vi "ZMQ Send command string input.vi"(4 "Int args":map{string, i32}(c390), 5 "String args":map{string, string}(c390), 6 "Bool args":map{string, bool}(c390), 7 "DBL args":map{string, dbl}(c390), 8 "error in":errorcluster, 9 "Command":string, 10 "Instrument":string, 11 "socket in":refnum<class "zmq_socket.lvclass">) -> (0 "error out":errorcluster, 1 "Standalone":bool, 2 "Recieved message":string=" INSTRUCTIONS:\r\rNormal Use:  When using subVIs that incorporate the error in/error out (or error I/O) structure, place this handler where you want to inform the user of an error, typically at the end of the I/O data path, as the last action of the program.  If the error in error? is ERROR, the handler creates a message describing the error and its source.  If the type of dialog = 1 (default), the message is displayed to the user, who can only acknowedge it.  If the type = 2, the user can acknowledge the message or abort execution; aborting a program with active I/O is not recommended.  If the type = 0, no message is displayed; this is used to process the error programmatically, and the error out cluster elements are wired to individual terminals for that reason.  \r\rOther Use:\n\r\nlocal testing.  To test the error code of a subVI or function that does not have the error I/O structure, you can wire its error code and a source string to the local error code and error source inputs.  If error in error? indicates no error and error code is not equal to 0, the local code and source are substituted for the error in values, and error? is set TRUE (ERROR).", 3 "socket out":refnum<class "zmq_socket.lvclass">)   [LabVIEW 2022 SP3]
uses:
  <vilib>/addons/zeromq/zmq_socket.lvclass
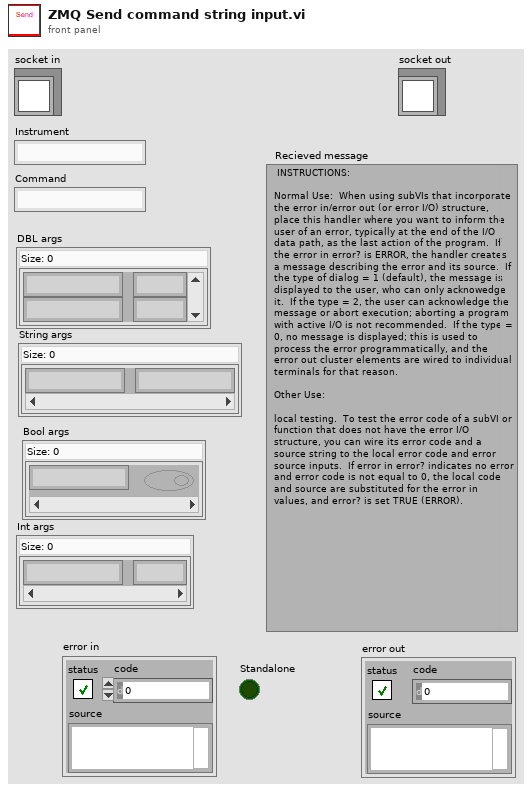
[diagram p1: front panel]
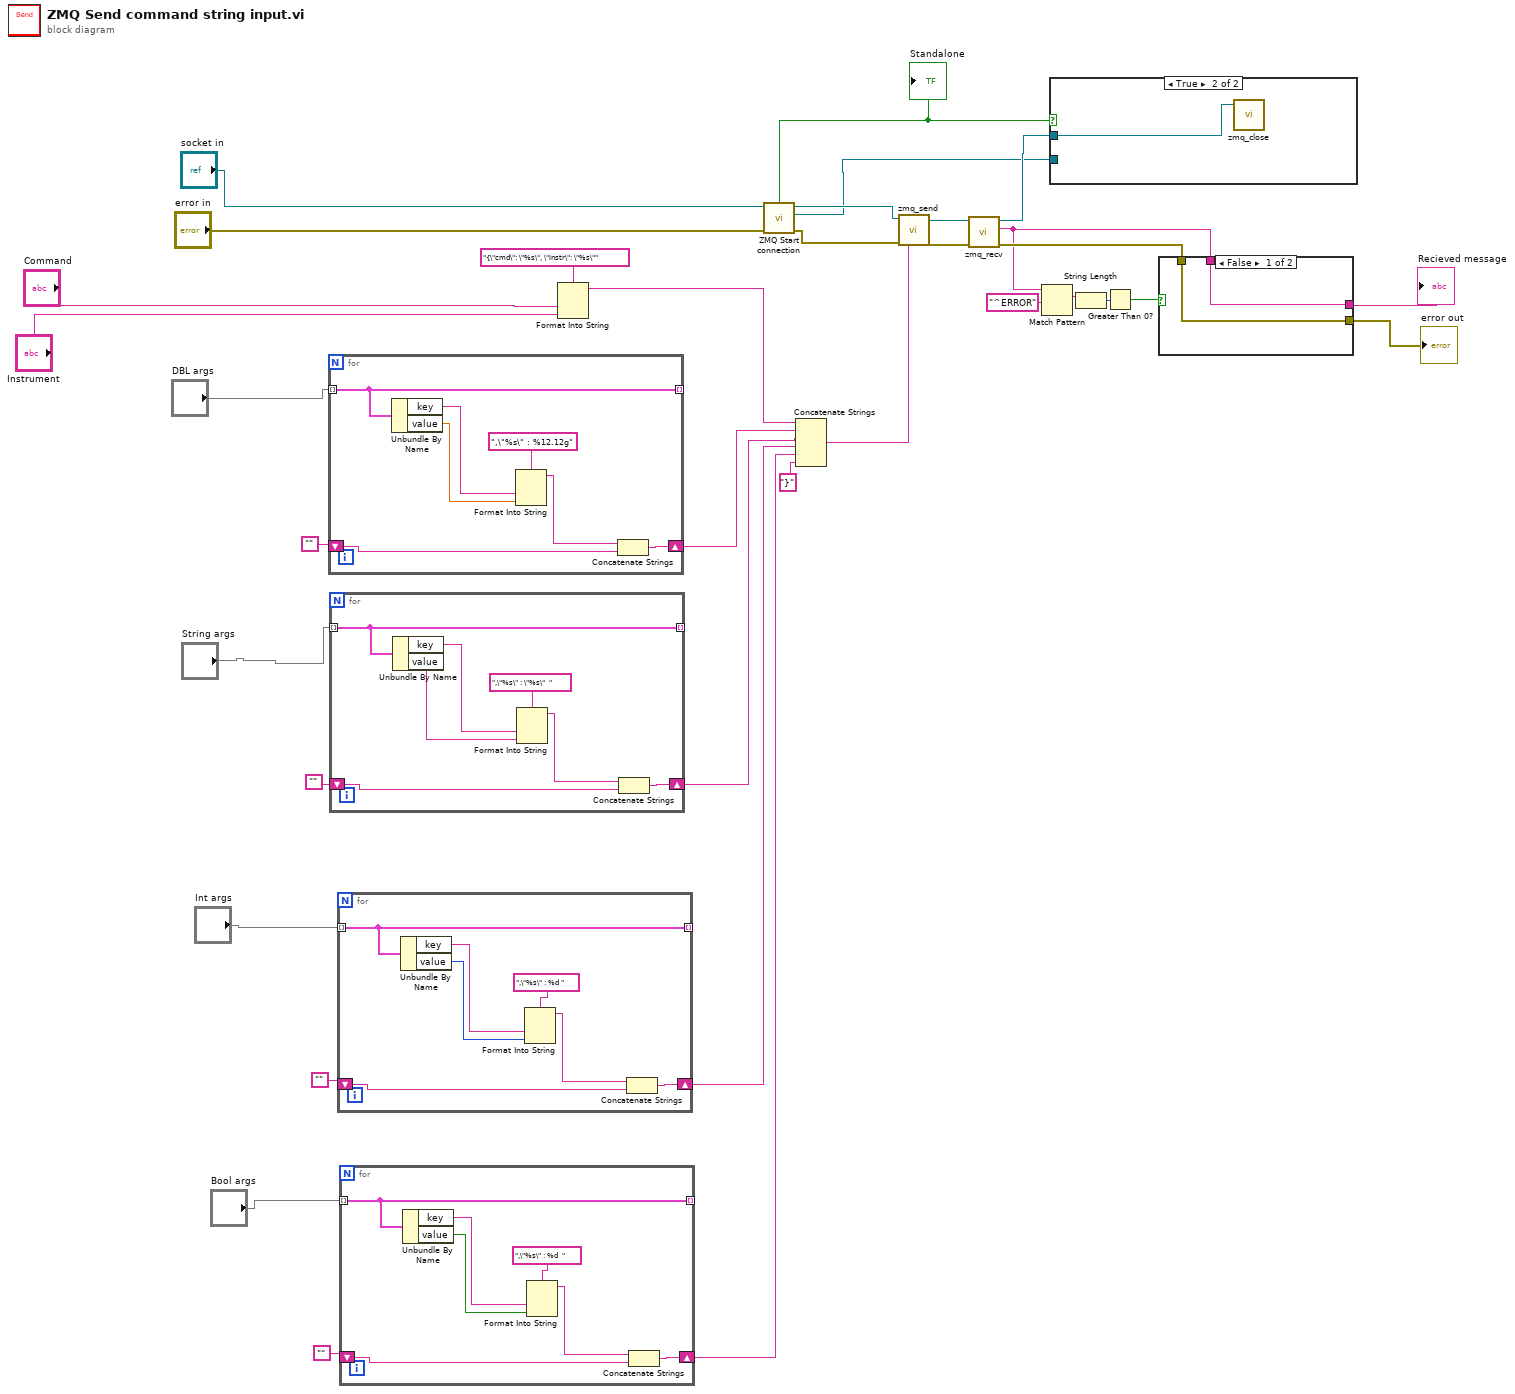
[diagram p0: block diagram]
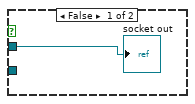
[diagram p2: hidden frame]
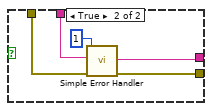
[diagram p3: hidden frame]
diagram:
  n1 = for {
    tunnel: [w41] -> _ mode=indexing
    tunnel: "DBL args" -> [w41] mode=indexing
    shift-right: [w38] -> w19
    shift-left: "" -> [w42]
    n2 = Unbundle By Name(w41) -> ("key"=w39:string, "value"=w40:dbl)
    n3 = Format Into String(format string=",\"%s\" : %12.12g", w39, w40) -> (resulting string=w36:string)  [unwired: 2 in, 1 out]
    n4 = Concatenate Strings(w36, w42) -> (w38:string)
  }
  n5 = for {
    tunnel: [w48] -> _ mode=indexing
    tunnel: "String args" -> [w48] mode=indexing
    shift-right: [w46] -> w12
    shift-left: "" -> [w49]
    n6 = Unbundle By Name(w48) -> ("key"=w47:string, "value"=w43:string)
    n7 = Format Into String(format string=",\"%s\" : \"%s\"  ", w47, w43) -> (resulting string=w44:string)  [unwired: 2 in, 1 out]
    n8 = Concatenate Strings(w44, w49) -> (w46:string)
  }
  n9 = for {
    tunnel: [w55] -> _ mode=indexing
    tunnel: "Int args" -> [w55] mode=indexing
    shift-right: [w53] -> w5
    shift-left: "" -> [w56]
    n10 = Unbundle By Name(w55) -> ("key"=w54:string, "value"=w50:i32)
    n11 = Format Into String(format string=",\"%s\" : %d ", w54, w50) -> (resulting string=w51:string)  [unwired: 2 in, 1 out]
    n12 = Concatenate Strings(w51, w56) -> (w53:string)
  }
  n13 = for {
    tunnel: [w62] -> _ mode=indexing
    tunnel: "Bool args" -> [w62] mode=indexing
    shift-right: [w60] -> w4
    shift-left: "" -> [w63]
    n14 = Unbundle By Name(w62) -> ("key"=w61:string, "value"=w57:bool)
    n15 = Format Into String(format string=",\"%s\" : %d  ", w61, w57) -> (resulting string=w58:string)  [unwired: 2 in, 1 out]
    n16 = Concatenate Strings(w58, w63) -> (w60:string)
  }
  n17 = Format Into String(format string="{\"cmd\": \"%s\", \"instr\": \"%s\"", "Command", "Instrument") -> (resulting string=w16:string)  [unwired: 2 in, 1 out]
  n18 = call "ZMQ Start connection.vi"("error in"="error in", "socket in"="socket in") -> ("error out"=w22:errorcluster, "Standalone"=w21:bool, "context out"=w1:refnum<class "zmq_context.lvclass">, "socket out"=w24:refnum<class "zmq_socket.lvclass">)  [unwired: 5 in]
  "Standalone" <- w21
  n19 = Concatenate Strings(w16, w19, w12, w5, w4, "}" ("string")) -> (w18:string)
  n20 = call <vilib>:"zmq_send.vi"("error in"=w22, "data"=w18, "socket in"=w24) -> ("error out"=w27:errorcluster, "socket out"=w26:refnum<class "zmq_socket.lvclass">)  [unwired: 4 in]
  n21 = call <vilib>:"zmq_recv.vi"("error in"=w27, "socket in"=w26) -> ("error out"=w34:errorcluster, "data"=w31:string, "socket out"=w20:refnum<class "zmq_socket.lvclass">)  [unwired: 3 in, 2 out]
  n22 = Match Pattern(string=w31, regular expression="^ERROR") -> (match substring=w29:string)  [unwired: 1 in, 3 out]
  n23 = case shown="True" w21 {
    tunnel: w20 -> [w64 w65]
    tunnel: w1 -> [_ _]
    frame False {
      "socket out" <- w64
    }
    frame True {
      n24 = call <vilib>:"zmq_close.vi"("socket"=w65) -> ()  [unwired: 4 in, 1 out]
    }
  }
  n25 = String Length(string=w29) -> (length=w30:i32)
  n26 = Greater Than 0?(x=w30) -> (x > 0?=w28:bool)
  n27 = case shown="False" w28 {
    tunnel: w34 -> [w67 w72]
    tunnel: [w67 w71] -> w33
    tunnel: [w66 w70] -> w32
    tunnel: w31 -> [w66 w68]
    frame False {
    }
    frame True {
      n28 = call <vilib>:"Simple Error Handler.vi"("error code (no error:0)"=1, "error source (\" \")"=w68, "error in (no error)"=w72) -> ("error out"=w71:errorcluster, "message"=w70:string)  [unwired: 2 in, 3 out]
    }
  }
  "Recieved message" <- w32
  "error out" <- w33
